vi "Insert into Subpanel.vi"(6 "SubPanel":refnum<vi>, 8 "error in (no error)":errorcluster, 9 "VI":refnum<vi>, 10 "Panel":refnum<class "Panel.lvclass">, 11 "Manager in":refnum<class "Manager.lvclass">) -> (0 "error out":errorcluster, 3 "Manager out":refnum<class "Manager.lvclass">)   [LabVIEW 2020, in "OOPanel.lvlib" / "Manager.lvclass"]
uses:
  Manager.lvclass
  Panel/Panel.lvclass
  Panel/Visibility State.ctl
  Manager.lvclass/Manager.ctl
  <vilib>/Utility/miscctls.llb/LVMapReplaceAction.ctl
  OOPanel.lvlib
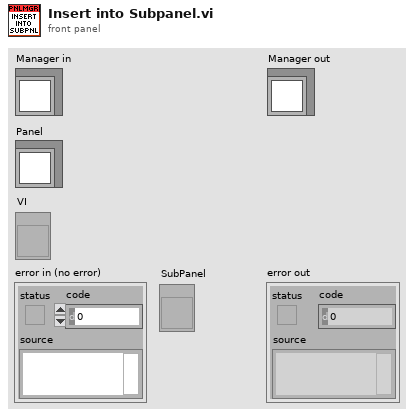
[diagram p1: front panel]
types:
  T1 = typedef "OOPanel.lvlib/Visibility State.ctl" = enum16{"Idle", "Closed", "Hidden", "Visible", "Subpanel"}
  T2 = typedef "LVMapReplaceAction.ctl" = enum32{"Modify Entry only if found", "Add or Modify Entry", "Delete Entry"}
  T3 = typedef "OOPanel.lvlib/Manager.lvclass/Ref Data.ctl" = cluster{"Created Panels":refnum<class "Panel.lvclass">[], "Subpanel Map":map{refnum<vi>, T4}}
  T4 = typedef "OOPanel.lvlib/Manager.lvclass/Subpanel Data.ctl" = cluster{"Panel":refnum<class "Panel.lvclass">, "Has Panel":bool, "Visible":bool}
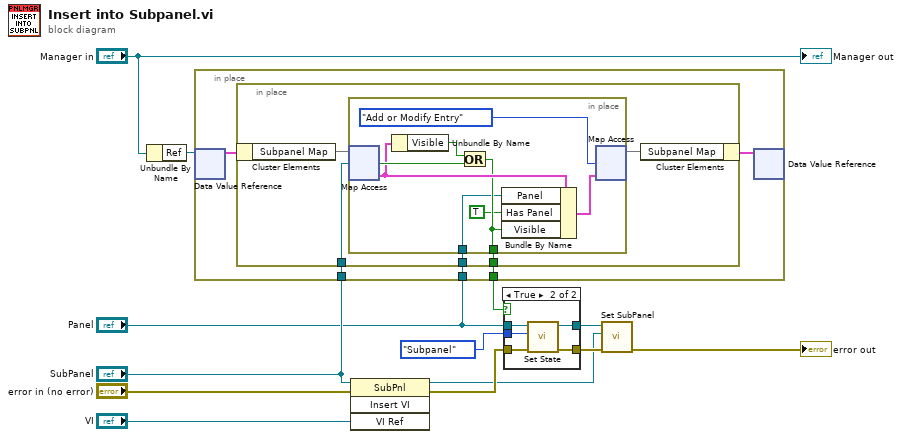
[diagram p0: block diagram]
diagram:
  n1 = Unbundle By Name("Manager in") -> ("Ref"=w12:refnum<data-value>)
  n2 = in-place {
    in-place-border: "SubPanel" -> [w16]
    in-place-border: [w15] -> w4
    in-place-border: "Panel" -> [w14]
    n3 = in-place-dvr #1(w12) -> (w18:T3)  [unwired: 1 out]
    n4 = in-place {
      in-place-border: w16 -> [w21]
      in-place-border: [w20] -> w15
      in-place-border: w14 -> [w19]
      n5 = in-place-cluster #2(w18) -> ("Subpanel Map"=w23:map{refnum<vi>, T4})
      n6 = in-place {
        in-place-border: [w26] -> w20
        in-place-border: w19 -> [w24]
        n7 = in-place-map #3(w23, w21) -> (w28:T4, w29:bool)  [unwired: 1 in]
        n8 = Unbundle By Name(w28) -> ("Visible"=w30:bool)
        n9 = Or(x=w30, y=w29) -> (x .or. y?=w26:bool)
        n10 = Bundle By Name(cluster=w28, "Panel"=w24, "Has Panel"=TRUE, "Visible"=w26) -> (w27:T4)
        n11 = in-place-map #3(w27, LVMapReplaceAction."Add or Modify Entry" ("action")) -> (w22:map{refnum<vi>, T4})  [unwired: 2 out]
      }
      n12 = in-place-cluster #2("Subpanel Map"=w22) -> (w17:T3)
    }
    n13 = in-place-dvr #1(w17) -> ()  [unwired: 2 out]
  }
  n14 = invoke class="SubPnl" method="Insert VI"(reference="SubPanel", error in="error in (no error)", "VI Ref"="VI") -> (reference out=w9:refnum<vi>, error out=w11:errorcluster)  [unwired: 1 in, 2 out]
  n15 = case shown="True" w4 {
    tunnel: [w32 w38] -> w13
    tunnel: w11 -> [w32 w37]
    tunnel: [w33 w36] -> w10
    tunnel: "Panel" -> [w33 w35]
    tunnel: Visibility_State."Subpanel" ("State") -> [_ w34]
    frame False {
    }
    frame True {
      n16 = call "Set State.vi"("error in (no error)"=w37, "State"=w34, "Panel in"=w35) -> ("error out"=w38:errorcluster, "Panel out"=w36:refnum<class "Panel.lvclass">)  [unwired: 7 in]
    }
  }
  n17 = call "Set SubPanel.vi"("error in (no error)"=w13, "SubPanel"=w9, "Panel in"=w10) -> ("error out"=→"error out":errorcluster)  [unwired: 7 in, 1 out]
  "Manager out" <- "Manager in"
